vi "Array Variant to Spreadsheet String.vi"(8 "error in (no error)":errorcluster, 11 "Array Variant":variant) -> (0 "error out":errorcluster, 2 "spreadsheet string":string, 3 "Array Variant  out (dup)":variant)   [LabVIEW 2020, in "Generic Config Handling.lvlib"]
doc: "This vi takes a variant which represents an array and converts it to a spreadsheet string.\n\nElements within rows are delineated by commas.\nRows are delineated by semicolons."
uses:
  Generic Config Handling.lvlib
  <vilib>/Utility/error.llb/whitespace.ctl
  <vilib>/Utility/VariantDataType/VariantType.lvlib
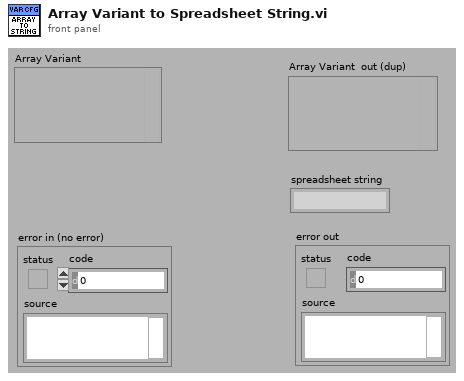
[diagram p1: front panel]
types:
  T1 = typedef "whitespace.ctl" = u16
  T2 = typedef "VariantType.lvlib/Type.ctl" = enum8{"Invalid Type", "Void", "I8", "I16", "I32", "I64", "U8", "U16", "U32", "U64", "Single Float", "Double Float", "Extended Float", "Single Complex", "Double Complex", "Extended Complex", "Enum U8", "Enum U16", "Enum U32", "Enum U64", "Single Float With Unit", "Double Float With Unit", "Extended Float With Unit", "Single Complex with Unit", "Double Complex with Unit", "Extended Complex with Unit", "Boolean", "String", "Path", "Picture", "Tag", "Array", "Cluster", "Variant", "LV Variant", "Waveform", "Timestamp", "Digital Waveform", "Digital Data", "ExpressData", "Refnum", "External Data", "VI", "Poly VI", "LabVIEW Class Instance", "Fixed Point"}
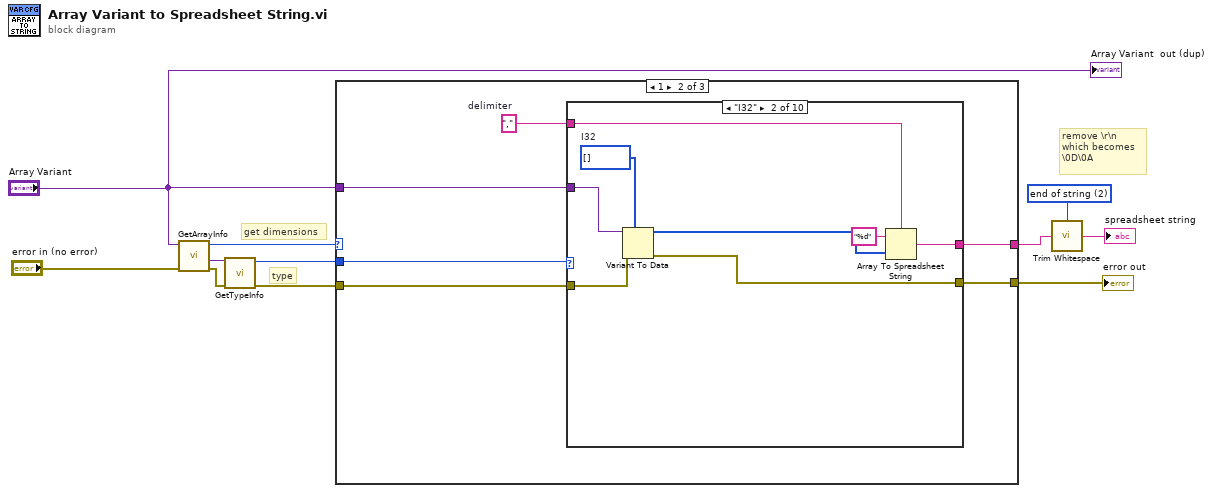
[diagram p0: block diagram]
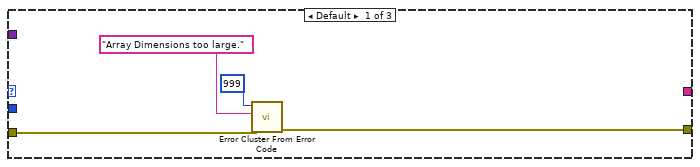
[diagram p2: hidden frame]
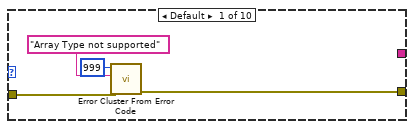
[diagram p3: hidden frame]
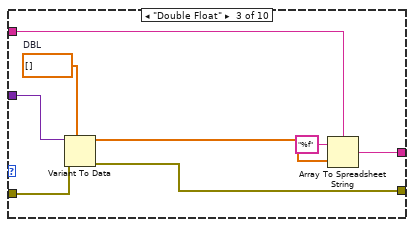
[diagram p4: hidden frame]
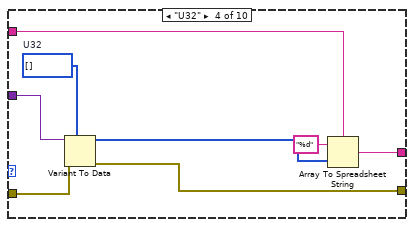
[diagram p5: hidden frame]
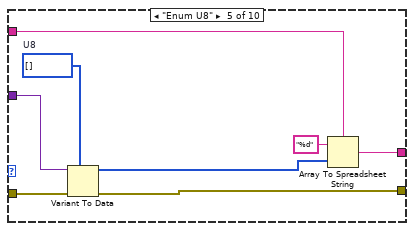
[diagram p6: hidden frame]
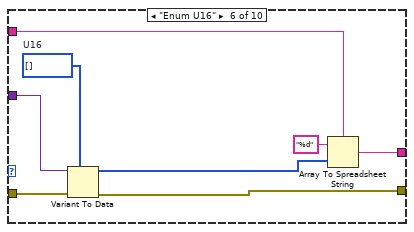
[diagram p7: hidden frame]
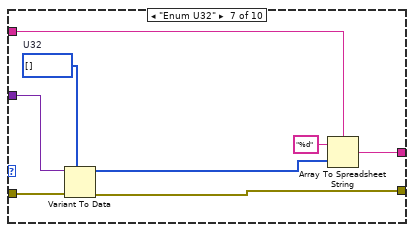
[diagram p8: hidden frame]
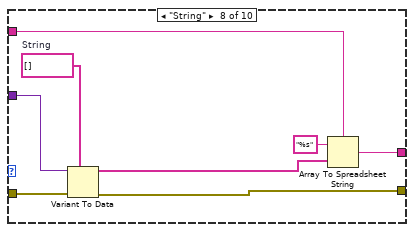
[diagram p9: hidden frame]
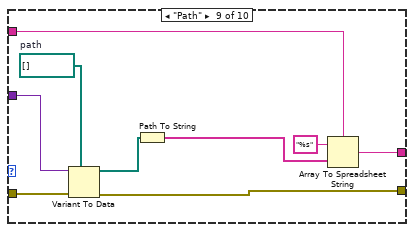
[diagram p10: hidden frame]
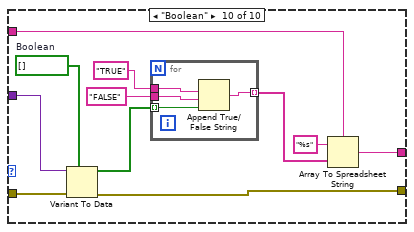
[diagram p11: hidden frame]
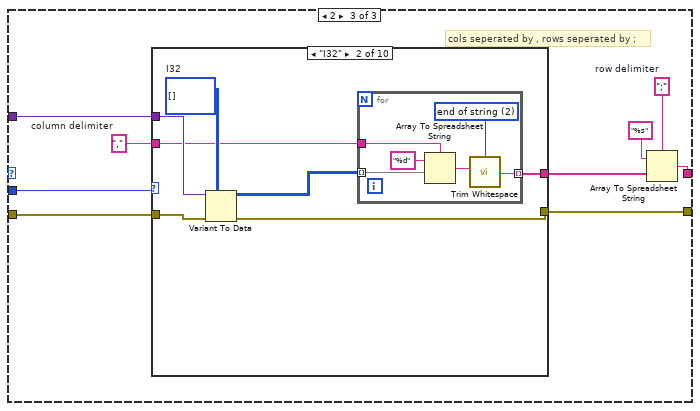
[diagram p12: hidden frame]
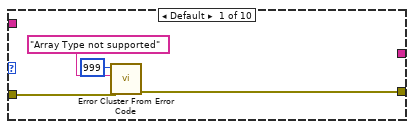
[diagram p13: hidden frame]
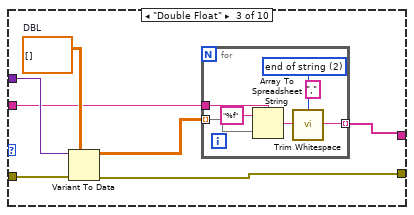
[diagram p14: hidden frame]
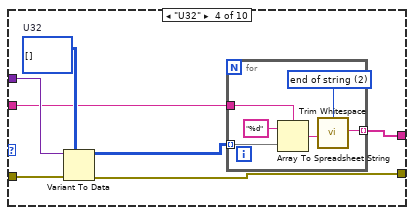
[diagram p15: hidden frame]
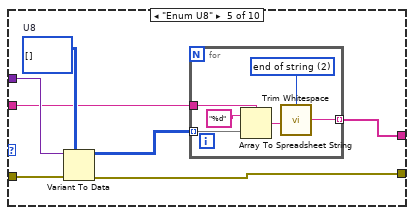
[diagram p16: hidden frame]
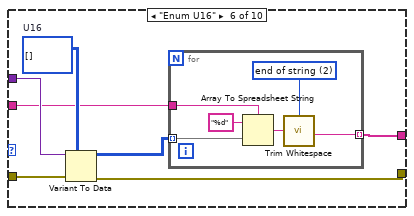
[diagram p17: hidden frame]
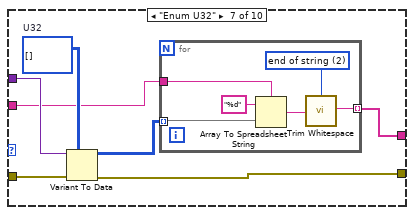
[diagram p18: hidden frame]
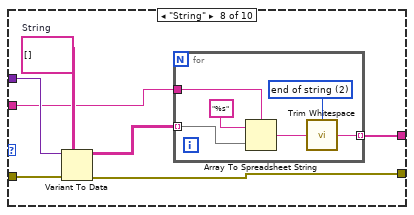
[diagram p19: hidden frame]
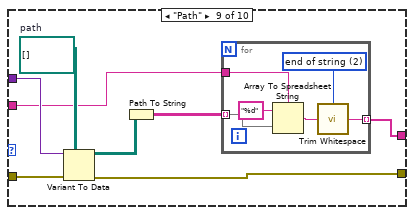
[diagram p20: hidden frame]
diagram:
  w3 = T1 2 items=["both", "start of string", "end of string"] ("location (both)")
  # "type"
  # "get dimensions"
  # "remove \\r\\n\nwhich becomes\n\\0D\\0A"
  n1 = call <vilib>:"GetArrayInfo.vi"("error in (no error)"="error in (no error)", "Variant"="Array Variant") -> ("error out"=w8:errorcluster, "ArrayElement"=w7:variant, "NDims"=w6:i32)  [unwired: 6 in, 1 out]
  n2 = call <vilib>:"GetTypeInfo.vi"("error in (no error)"=w8, "Variant"=w7) -> ("error out"=w11:errorcluster, "Type Enum"=w9:T2)  [unwired: 5 in, 3 out]
  n3 = case shown="1" w6 {
    tunnel: w11 -> [w13 w18 w112]
    tunnel: [w12 w20 w113] -> w5
    tunnel: "Array Variant" -> [_ w17 w111]
    tunnel: w9 -> [_ w21 w114]
    tunnel: [_ w19 w107] -> w2
    frame Default {
      n4 = call <vilib>:"Error Cluster From Error Code.vi"("error in (no error)"=w13, "error message (\"\")"="Array Dimensions too large." ("error message (\"\")"), "error code (0)"=999) -> ("error out"=w12:errorcluster)  [unwired: 6 in]
    }
    frame 1 {
      w16 = ","  # delimiter
      n5 = case shown="\"I32\"" w21 {
        tunnel: [w23 w31 w39 w47 w55 w63 w71 w79 w88 w99] -> w20
        tunnel: [_ w33 w41 w49 w57 w65 w73 w81 w90 w101] -> w19
        tunnel: w18 -> [w22 w32 w40 w48 w56 w64 w72 w80 w89 w100]
        tunnel: w17 -> [_ w30 w38 w46 w54 w62 w70 w78 w87 w98]
        tunnel: w16 -> [_ w26 w34 w42 w50 w58 w66 w74 w82 w91]
        frame Default {
          n6 = call <vilib>:"Error Cluster From Error Code.vi"("error in (no error)"=w22, "error message (\"\")"="Array Type not supported" ("error message (\"\")"), "error code (0)"=999) -> ("error out"=w23:errorcluster)  [unwired: 6 in]
        }
        frame "I32" {
          w29 = i32[] []  # I32
          n7 = Variant To Data(error in=w32, type=w29, Variant=w30) -> (data=w28:i32[], error out=w31:errorcluster)
          n8 = Array To Spreadsheet String(delimiter (Tab)=w26, array=w28, 3:"%d" ("format string")) -> (spreadsheet string=w33:string)
        }
        frame "Double Float" {
          w37 = dbl[] []  # DBL
          n9 = Variant To Data(error in=w40, type=w37, Variant=w38) -> (data=w36:dbl[], error out=w39:errorcluster)
          n10 = Array To Spreadsheet String(delimiter (Tab)=w34, array=w36, 3:"%f" ("format string")) -> (spreadsheet string=w41:string)
        }
        frame "U32" {
          w45 = u32[] []  # U32
          n11 = Variant To Data(error in=w48, type=w45, Variant=w46) -> (data=w44:u32[], error out=w47:errorcluster)
          n12 = Array To Spreadsheet String(delimiter (Tab)=w42, array=w44, 3:"%d" ("format string")) -> (spreadsheet string=w49:string)
        }
        frame "Enum U8" {
          w53 = u8[] []  # U8
          n13 = Variant To Data(error in=w56, type=w53, Variant=w54) -> (data=w52:u8[], error out=w55:errorcluster)
          n14 = Array To Spreadsheet String(delimiter (Tab)=w50, array=w52, 3:"%d" ("format string")) -> (spreadsheet string=w57:string)
        }
        frame "Enum U16" {
          w61 = u16[] []  # U16
          n15 = Variant To Data(error in=w64, type=w61, Variant=w62) -> (data=w60:u16[], error out=w63:errorcluster)
          n16 = Array To Spreadsheet String(delimiter (Tab)=w58, array=w60, 3:"%d" ("format string")) -> (spreadsheet string=w65:string)
        }
        frame "Enum U32" {
          w69 = u32[] []  # U32
          n17 = Variant To Data(error in=w72, type=w69, Variant=w70) -> (data=w68:u32[], error out=w71:errorcluster)
          n18 = Array To Spreadsheet String(delimiter (Tab)=w66, array=w68, 3:"%d" ("format string")) -> (spreadsheet string=w73:string)
        }
        frame "String" {
          w77 = string[] []  # String
          n19 = Variant To Data(error in=w80, type=w77, Variant=w78) -> (data=w75:string[], error out=w79:errorcluster)
          n20 = Array To Spreadsheet String(delimiter (Tab)=w74, array=w75, 3:"%s" ("format string")) -> (spreadsheet string=w81:string)
        }
        frame "Path" {
          w86 = path[] []  # path
          n21 = Variant To Data(error in=w89, type=w86, Variant=w87) -> (data=w84:path[], error out=w88:errorcluster)
          n22 = Path To String(path=w84) -> (string=w83:string[])
          n23 = Array To Spreadsheet String(delimiter (Tab)=w82, array=w83, 3:"%s" ("format string")) -> (spreadsheet string=w90:string)
        }
        frame "Boolean" {
          w97 = bool[] []  # Boolean
          n24 = Variant To Data(error in=w100, type=w97, Variant=w98) -> (data=w95:bool[], error out=w99:errorcluster)
          n25 = for {
            tunnel: w95 -> [w105] mode=indexing
            tunnel: "TRUE" ("string (\"\")") -> [w104]
            tunnel: "FALSE" ("false string") -> [w103]
            tunnel: [w102] -> w92 mode=indexing
            n26 = Append True/False String(1:w105, 2:w103, 3:w104) -> (0:w102:string)  [unwired: 1 in]
          }
          n27 = Array To Spreadsheet String(delimiter (Tab)=w91, array=w92, 3:"%s" ("format string")) -> (spreadsheet string=w101:string)
        }
      }
    }
    frame 2 {
      w106 = ","  # column delimiter
      w109 = ";"  # row delimiter
      # "cols seperated by , rows seperated by ;"
      n28 = case shown="\"I32\"" w114 {
        tunnel: [w116 w123 w137 w150 w163 w176 w189 w202 w216 w232] -> w113
        tunnel: [_ w125 w133 w146 w159 w172 w185 w198 w213 w225] -> w108
        tunnel: w112 -> [w115 w124 w138 w151 w164 w177 w190 w203 w217 w233]
        tunnel: w111 -> [_ w122 w136 w149 w162 w175 w188 w201 w215 w231]
        tunnel: w106 -> [_ w119 w132 w145 w158 w171 w184 w197 w210 w224]
        frame Default {
          n29 = call <vilib>:"Error Cluster From Error Code.vi"("error in (no error)"=w115, "error message (\"\")"="Array Type not supported" ("error message (\"\")"), "error code (0)"=999) -> ("error out"=w116:errorcluster)  [unwired: 6 in]
        }
        frame "I32" {
          w121 = i32[][] []  # I32
          n30 = Variant To Data(error in=w124, type=w121, Variant=w122) -> (data=w120:i32[][], error out=w123:errorcluster)
          n31 = for {
            tunnel: [w128] -> w125 mode=indexing
            tunnel: w120 -> [w127] mode=indexing
            tunnel: w119 -> [w126]
            w130 = T1 2 items=["both", "start of string", "end of string"] ("location (both)")
            n32 = Array To Spreadsheet String(delimiter (Tab)=w126, array=w127, 3:"%d" ("format string")) -> (spreadsheet string=w129:string)
            n33 = call <vilib>:"Trim Whitespace.vi"("string"=w129, "location (both)"=w130) -> ("trimmed string"=w128:string)
          }
        }
        frame "Double Float" {
          (unwired) "," ("delimiter (Tab)")
          w135 = dbl[][] []  # DBL
          n34 = Variant To Data(error in=w138, type=w135, Variant=w136) -> (data=w134:dbl[][], error out=w137:errorcluster)
          n35 = for {
            tunnel: [w140] -> w133 mode=indexing
            tunnel: w134 -> [w144] mode=indexing
            tunnel: w132 -> [w139]
            w142 = T1 2 items=["both", "start of string", "end of string"] ("location (both)")
            n36 = Array To Spreadsheet String(delimiter (Tab)=w139, array=w144, 3:"%f" ("format string")) -> (spreadsheet string=w141:string)
            n37 = call <vilib>:"Trim Whitespace.vi"("string"=w141, "location (both)"=w142) -> ("trimmed string"=w140:string)
          }
        }
        frame "U32" {
          w148 = u32[][] []  # U32
          n38 = Variant To Data(error in=w151, type=w148, Variant=w149) -> (data=w147:u32[][], error out=w150:errorcluster)
          n39 = for {
            tunnel: [w153] -> w146 mode=indexing
            tunnel: w147 -> [w157] mode=indexing
            tunnel: w145 -> [w152]
            w155 = T1 2 items=["both", "start of string", "end of string"] ("location (both)")
            n40 = Array To Spreadsheet String(delimiter (Tab)=w152, array=w157, 3:"%d" ("format string")) -> (spreadsheet string=w154:string)
            n41 = call <vilib>:"Trim Whitespace.vi"("string"=w154, "location (both)"=w155) -> ("trimmed string"=w153:string)
          }
        }
        frame "Enum U8" {
          w161 = u8[][] []  # U8
          n42 = Variant To Data(error in=w164, type=w161, Variant=w162) -> (data=w160:u8[][], error out=w163:errorcluster)
          n43 = for {
            tunnel: [w166] -> w159 mode=indexing
            tunnel: w160 -> [w170] mode=indexing
            tunnel: w158 -> [w165]
            w168 = T1 2 items=["both", "start of string", "end of string"] ("location (both)")
            n44 = Array To Spreadsheet String(delimiter (Tab)=w165, array=w170, 3:"%d" ("format string")) -> (spreadsheet string=w167:string)
            n45 = call <vilib>:"Trim Whitespace.vi"("string"=w167, "location (both)"=w168) -> ("trimmed string"=w166:string)
          }
        }
        frame "Enum U16" {
          w174 = u16[][] []  # U16
          n46 = Variant To Data(error in=w177, type=w174, Variant=w175) -> (data=w173:u16[][], error out=w176:errorcluster)
          n47 = for {
            tunnel: [w179] -> w172 mode=indexing
            tunnel: w173 -> [w183] mode=indexing
            tunnel: w171 -> [w178]
            w181 = T1 2 items=["both", "start of string", "end of string"] ("location (both)")
            n48 = Array To Spreadsheet String(delimiter (Tab)=w178, array=w183, 3:"%d" ("format string")) -> (spreadsheet string=w180:string)
            n49 = call <vilib>:"Trim Whitespace.vi"("string"=w180, "location (both)"=w181) -> ("trimmed string"=w179:string)
          }
        }
        frame "Enum U32" {
          w187 = u32[][] []  # U32
          n50 = Variant To Data(error in=w190, type=w187, Variant=w188) -> (data=w186:u32[][], error out=w189:errorcluster)
          n51 = for {
            tunnel: [w192] -> w185 mode=indexing
            tunnel: w186 -> [w196] mode=indexing
            tunnel: w184 -> [w191]
            w194 = T1 2 items=["both", "start of string", "end of string"] ("location (both)")
            n52 = Array To Spreadsheet String(delimiter (Tab)=w191, array=w196, 3:"%d" ("format string")) -> (spreadsheet string=w193:string)
            n53 = call <vilib>:"Trim Whitespace.vi"("string"=w193, "location (both)"=w194) -> ("trimmed string"=w192:string)
          }
        }
        frame "String" {
          w200 = string[][] []  # String
          n54 = Variant To Data(error in=w203, type=w200, Variant=w201) -> (data=w199:string[][], error out=w202:errorcluster)
          n55 = for {
            tunnel: [w205] -> w198 mode=indexing
            tunnel: w199 -> [w208] mode=indexing
            tunnel: w197 -> [w204]
            w207 = T1 2 items=["both", "start of string", "end of string"] ("location (both)")
            n56 = Array To Spreadsheet String(delimiter (Tab)=w204, array=w208, 3:"%s" ("format string")) -> (spreadsheet string=w206:string)
            n57 = call <vilib>:"Trim Whitespace.vi"("string"=w206, "location (both)"=w207) -> ("trimmed string"=w205:string)
          }
        }
        frame "Path" {
          w214 = path[][] []  # path
          n58 = Variant To Data(error in=w217, type=w214, Variant=w215) -> (data=w212:path[][], error out=w216:errorcluster)
          n59 = Path To String(path=w212) -> (string=w211:string[][])
          n60 = for {
            tunnel: [w219] -> w213 mode=indexing
            tunnel: w211 -> [w223] mode=indexing
            tunnel: w210 -> [w218]
            w221 = T1 2 items=["both", "start of string", "end of string"] ("location (both)")
            n61 = Array To Spreadsheet String(delimiter (Tab)=w218, array=w223, 3:"%d" ("format string")) -> (spreadsheet string=w220:string)
            n62 = call <vilib>:"Trim Whitespace.vi"("string"=w220, "location (both)"=w221) -> ("trimmed string"=w219:string)
          }
        }
        frame "Boolean" {
          w230 = bool[][] []  # Boolean
          n63 = Variant To Data(error in=w233, type=w230, Variant=w231) -> (data=w229:bool[][], error out=w232:errorcluster)
          n64 = for {
            tunnel: w229 -> [w243] mode=indexing
            tunnel: "TRUE" ("string (\"\")") -> [w242]
            tunnel: "FALSE" ("false string") -> [w241]
            tunnel: [w240] -> w226 mode=indexing
            n65 = for {
              tunnel: w243 -> [w247] mode=indexing
              tunnel: w242 -> [w246]
              tunnel: w241 -> [w245]
              tunnel: [w244] -> w240 mode=indexing
              n66 = Append True/False String(1:w247, 2:w245, 3:w246) -> (0:w244:string)  [unwired: 1 in]
            }
          }
          n67 = for {
            tunnel: [w235] -> w225 mode=indexing
            tunnel: w226 -> [w238] mode=indexing
            tunnel: w224 -> [w234]
            w237 = T1 2 items=["both", "start of string", "end of string"] ("location (both)")
            n68 = Array To Spreadsheet String(delimiter (Tab)=w234, array=w238, 3:"%s" ("format string")) -> (spreadsheet string=w236:string)
            n69 = call <vilib>:"Trim Whitespace.vi"("string"=w236, "location (both)"=w237) -> ("trimmed string"=w235:string)
          }
        }
      }
      n70 = Array To Spreadsheet String(delimiter (Tab)=w109, array=w108, 3:"%s" ("format string")) -> (spreadsheet string=w107:string)
    }
  }
  "error out" <- w5
  n71 = call <vilib>:"Trim Whitespace.vi"("string"=w2, "location (both)"=w3) -> ("trimmed string"=→"spreadsheet string":string)
  "Array Variant  out (dup)" <- "Array Variant"
